vi "Read Time Scale.vi"(8 "error in (no error)":errorcluster, 11 "Worker In":refnum<class "Worker.lvclass">) -> (0 "error out":errorcluster, 2 "Time Scale [ms]":u32, 3 "Worker Out":refnum<class "Worker.lvclass">)   [LabVIEW 2020, in "Worker.lvclass"]
uses:
  Worker.lvclass
  Worker.lvclass/Worker.ctl
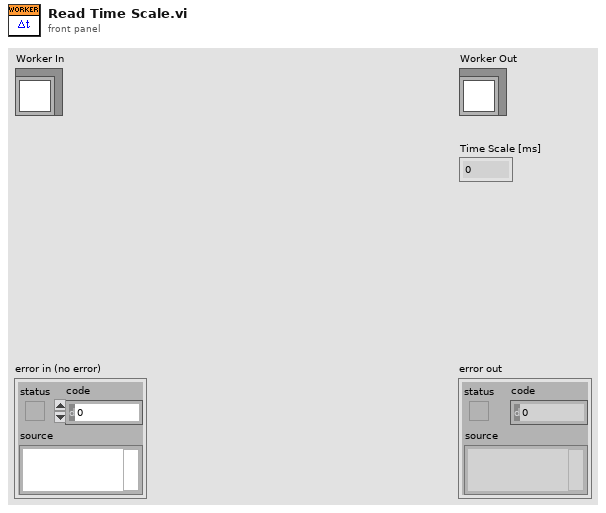
[diagram p1: front panel]
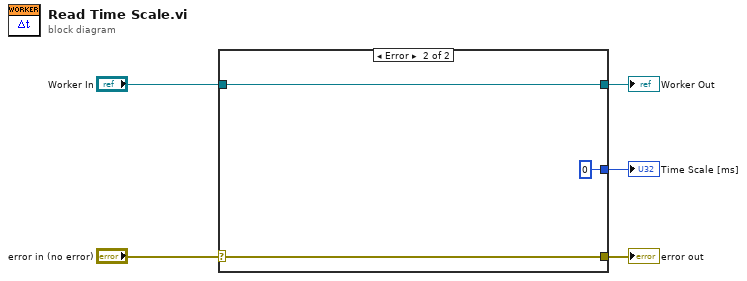
[diagram p0: block diagram]
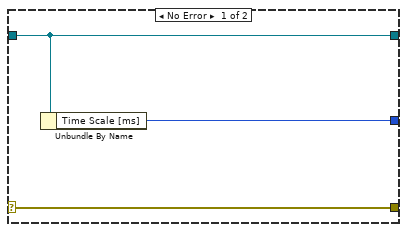
[diagram p2: hidden frame]
diagram:
  n1 = case shown="Error" "error in (no error)" {
    selector: "error in (no error)" -> [w8 w10]
    tunnel: [w8 w10] -> w4
    tunnel: [w7 w11] -> w2
    tunnel: "Worker In" -> [w7 w11]
    tunnel: [w6 u32 0 ("Time Scale [ms]")] -> w1
    frame No Error {
      n2 = Unbundle By Name(w7) -> ("Time Scale [ms]"=w6:u32)
    }
    frame Error {
    }
  }
  "error out" <- w4
  "Worker Out" <- w2
  "Time Scale [ms]" <- w1
